vi "GetTrueString.vi"(10 "BoolArray":bool[](array[boolean]), 11 "StrArray":string[](array[string])) -> (7 "TrueArray":string[](array[string]))   [LabVIEW 2014]
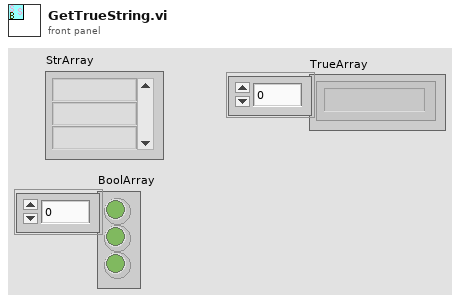
[diagram p1: front panel]
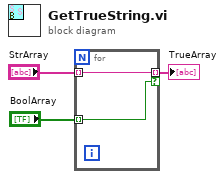
[diagram p0: block diagram]
diagram:
  n1 = for {
    tunnel: "StrArray" -> [w5] mode=indexing
    tunnel: "BoolArray" -> [w4] mode=indexing
    tunnel: [w5] -> w1 mode=indexing if=w4
  }
  "TrueArray" <- w1
